vi "Init Device.vi"(8 "error in (no error)":errorcluster, 11 "Synchronization Device in":refnum<class "Synchronization Device.lvclass">) -> (0 "error out":errorcluster, 3 "Synchronization Device out":refnum<class "Synchronization Device.lvclass">)   [LabVIEW 2015, in "Synchronization Device.lvlib" / "Synchronization Device.lvclass"]
uses:
  Synchronization Device.lvclass
  Device/Device.lvclass
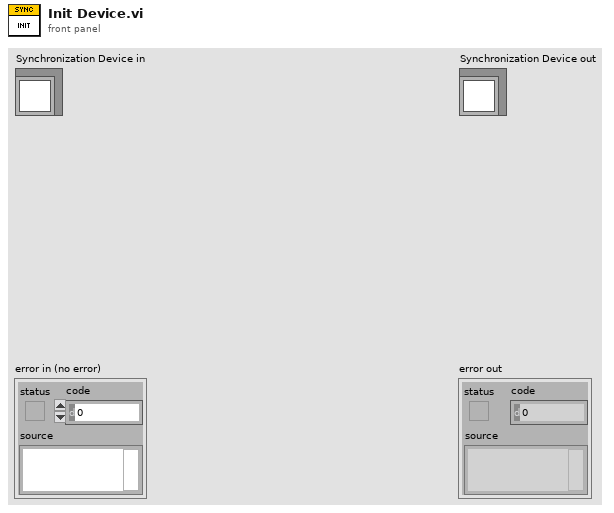
[diagram p1: front panel]
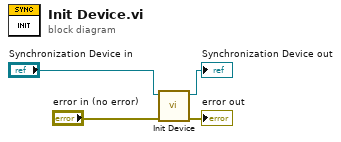
[diagram p0: block diagram]
diagram:
  n1 = call-parent "Init Device.vi"("error in (no error)"="error in (no error)", "Device in"="Synchronization Device in") -> ("error out"=→"error out":errorcluster, "Device out"=→"Synchronization Device out":refnum<class "Synchronization Device.lvclass">)  [unwired: 8 in]
